vi "Grid_num_der.vi"(8 "error in (no error)":errorcluster, 9 "Settings":T1={"Cutoff frq I/V"=0.125, "Cutoff frq dI/dV"=0.125, "Filter order dI/DV"=2, "Filter type  dI/dV"=enum."Gaussian", "Filter order I/V"=2, "Filter type I/V"=enum."Gaussian"} {"Filter order I/V" min=1 max=1000 step=1; "Filter order dI/DV" min=1 max=1000 step=1}, 11 "Binary Spectroscopy File":path) -> (0 "error out":errorcluster)   [LabVIEW 2021]
uses:
  <userlib>/Nanonis Prog Interface V5/Nanonis Prog Interface.lvlib
panel:
  out "error out Write file":errorcluster
  out "error out Read file":errorcluster
  out "Progress":u8(slide) scale=0.0..100.0
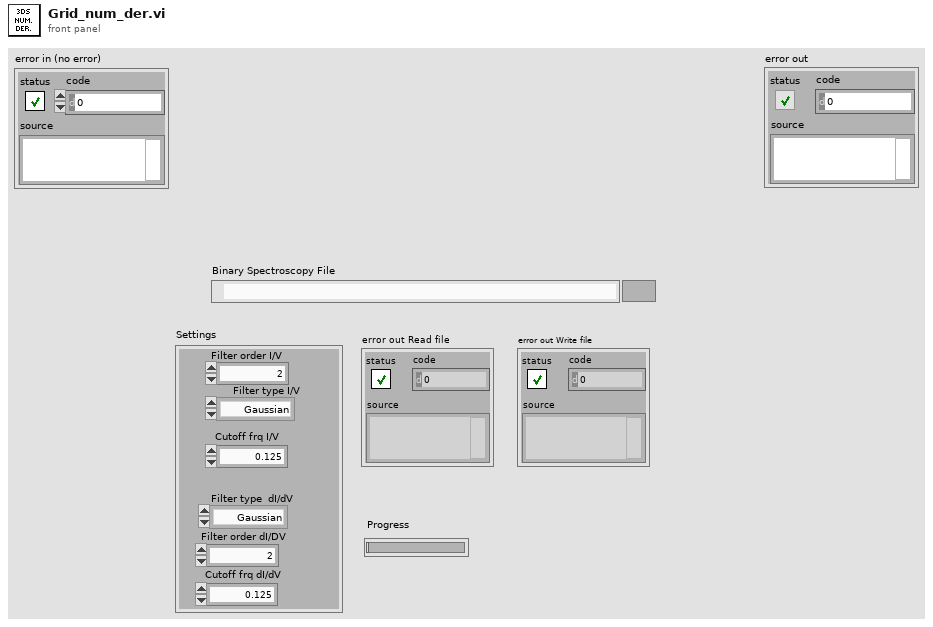
[diagram p1: front panel]
types:
  T1 = cluster{"Cutoff frq I/V":dbl, "Cutoff frq dI/dV":dbl, "Filter order dI/DV":i32, "Filter type  dI/dV":enum16{"none", "Gaussian", "Butterworth", "5th order FIR"}, "Filter order I/V":i32, "Filter type I/V":enum16{"none", "Gaussian", "Butterworth", "5th order FIR"}}
  T2 = typedef "Nanonis Prog Interface.lvlib/Binary_SpectroscopyFile-Config.ctl" = cluster{"Num Par":i32, "Exp size":i32, "Points":i32, "Grid Dim X":i32, "Grid Dim Y":i32, "Header size":i32, "Channels":string[], "Parameters":string[], "Sweep Signal":string, "Grid":cluster{"center X (m)":sgl, "center Y (m)":sgl, "width (m)":sgl, "height (m)":sgl, "angle (deg)":sgl}}
  T3 = cluster{"center X (m)":sgl, "center Y (m)":sgl, "width (m)":sgl, "height (m)":sgl, "angle (deg)":sgl}
  T4 = enum16{"none", "Gaussian", "Butterworth", "5th order FIR"}
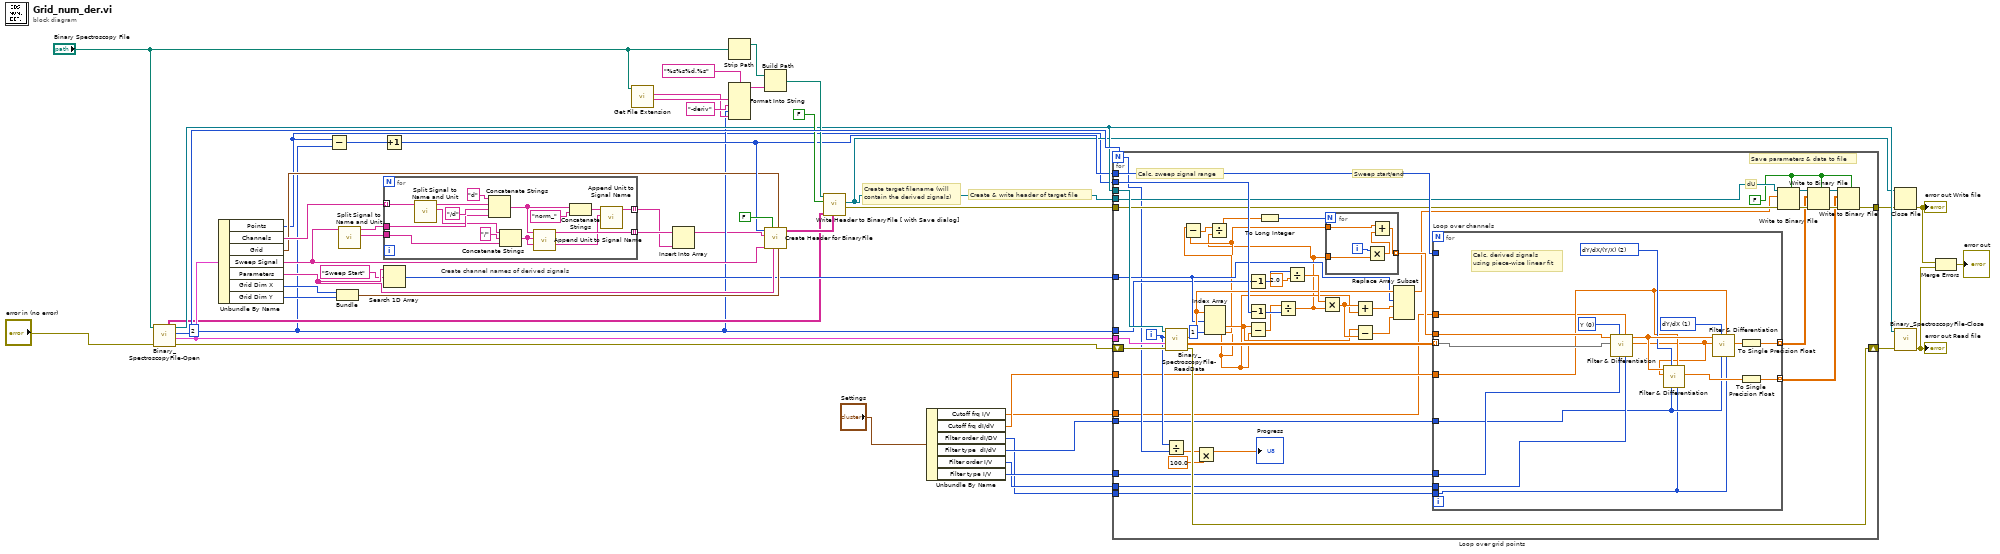
[diagram p0: block diagram]
diagram:
  w16 = u16 2 ("Fit length for derivative")
  # "Create & write header of target file"
  # "Create target filename (will contain the derived signals)"
  n1 = call <userlib>:"Binary_SpectroscopyFile-Open.vi"("error in (no error)"="error in (no error)", "Binary Spectroscopy File"="Binary Spectroscopy File") -> ("error out"=w48:errorcluster, "Config"=w36:T2, "Number of Experiments"=w49:i32, "File ref"=w37:refnum<file>, "Global Attributes"=w22:string[][])  [unwired: 5 in]
  n2 = Unbundle By Name(w36) -> ("Points"=w12:i32, "Channels"=w35:string[], "Grid"=w26:T3, "Sweep Signal"=w34:string, "Parameters"=w30:string[], "Grid Dim X"=w46:i32, "Grid Dim Y"=w45:i32)
  n3 = Subtract(x=w12, y=w16) -> (x-y=w31:i32)
  n4 = Bundle("Grid Dim X"=w46, "Grid Dim Y"=w45) -> (w44:cluster{"Grid Dim X":i32, "Grid Dim Y":i32})  [unwired: 1 in]
  n5 = call <userlib>:"Split Signal to Name and Unit.vi"("Name with unit"=w34) -> ("Unit"=w32:string, "Name"=w33:string)  [unwired: 5 in]
  n6 = Increment(x=w31) -> (x+1=w27:i32)
  n7 = for "Create channel names of derived signals" {
    tunnel: w35 -> [w63] mode=indexing
    tunnel: w33 -> [w59]
    tunnel: w32 -> [w56]
    tunnel: [w55] -> w14 mode=indexing
    tunnel: [w50] -> w13 mode=indexing
    n8 = call <userlib>:"Split Signal to Name and Unit.vi"("Name with unit"=w63) -> ("Unit"=w58:string, "Name"=w62:string)  [unwired: 5 in]
    n9 = Concatenate Strings("d" ("string"), w62, "/d" ("string"), w59) -> (w53:string)
    n10 = Concatenate Strings(w58, "/" ("string"), w56) -> (w54:string)
    n11 = call <userlib>:"Append Unit to Signal Name.vi"("Unit"=w54, "Name"=w53) -> ("Name with unit"=w55:string)  [unwired: 5 in]
    n12 = Concatenate Strings(w53, "norm_" ("string")) -> (w52:string)
    n13 = call <userlib>:"Append Unit to Signal Name.vi"("Unit"=w54, "Name"=w52) -> ("Name with unit"=w50:string)  [unwired: 5 in]
  }
  n14 = Search 1D Array(1D array=w30, element="Sweep Start") -> (index of element=w28:i32)  [unwired: 1 in]
  n15 = call <vilib>:"Get File Extension.vi"("file"="Binary Spectroscopy File") -> ("filename without extension"=w19:string, "lowercase file extension"=w18:string)  [unwired: 6 in, 3 out]
  n16 = Insert Into Array(array=w14, new element=w13) -> (w15:string[])  [unwired: 1 in]
  n17 = Strip Path(path="Binary Spectroscopy File") -> (stripped path=w42:path)  [unwired: 1 out]
  n18 = Format Into String(format string="%s%s%d.%s", w19, "-deriv" ("string"), w16, w18) -> (resulting string=w17:string)  [unwired: 2 in, 1 out]
  n19 = Build Path(base path=w42, name or relative path=w17) -> (appended path=w41:path)
  n20 = call <userlib>:"Create Header for BinaryFile.vi"("Grid points"=w44, "Grid param"=w26, "Fixed parameters"=w30, "Backward sweep"=FALSE, "Sweep signal"=w34, "Channels"=w15, "Points per sweep"=w27) -> ("Header (fixed attributes)"=w39:string[][])  [unwired: 4 in]
  n21 = call <userlib>:"Write Header to BinaryFile [ with Save dialog].vi"("Fixed Attributes"=w39, "Attributes in"=w22, "Show Dialog? (T)"=FALSE, "Filename"=w41) -> ("Error out"=w25:errorcluster, "File ref"=w23:refnum<file>)  [unwired: 4 in, 2 out]
  n22 = Unbundle By Name("Settings") -> ("Cutoff frq I/V"=w9:dbl, "Cutoff frq dI/dV"=w10:dbl, "Filter order dI/DV"=w5:i32, "Filter type  dI/dV"=w6:T4, "Filter order I/V"=w7:i32, "Filter type I/V"=w8:T4)
  n23 = for "Loop over grid points" {
    N: w49 -> [w72]
    tunnel: w37 -> [w112]
    tunnel: w36 -> [w111]
    shift-right: [w109] -> w38
    shift-left: w48 -> [w110]
    tunnel: w23 -> [w95]
    tunnel: w16 -> [w84]
    tunnel: w28 -> [w100]
    tunnel: w12 -> [w108]
    tunnel: w27 -> [w97]
    tunnel: w25 -> [w94]
    tunnel: [w91] -> w24
    tunnel: w10 -> [w69]
    tunnel: w9 -> [w68]
    tunnel: w8 -> [w67]
    tunnel: w7 -> [w66]
    tunnel: w6 -> [w65]
    tunnel: w5 -> [w64]
    i -> [w73]
    w88 = FALSE ("prepend array or string size? (T)")
    # "dU"
    # "Sweep start/end"
    # "Save parameters & data to file"
    # "Calc. sweep signal range"
    n24 = call <userlib>:"Binary_SpectroscopyFile-ReadData.vi"("error in"=w110, "Config"=w111, "Experiment to read (Index)"=w73, "File ref In"=w112) -> ("error out"=w109:errorcluster, "data"=w86:sgl[][], "Parameter values"=w101:sgl[])  [unwired: 4 in, 1 out]
    n25 = Divide(x=w73, y=w72) -> (x/y=w74:dbl)
    n26 = Multiply(x=w74, y=100.0) -> (x*y=→"Progress":dbl)
    n27 = Index Array(array=w101, index #1=w100, index #3=1 ("index")) -> (element #1=w79:sgl, element #2=w82:sgl, element #3=w80:sgl)  [unwired: 1 in]
    n28 = Subtract(x=w80, y=w79) -> (x-y=w78:sgl)
    n29 = Decrement(x=w84) -> (x-1=w105:u16)
    n30 = Decrement(x=w108) -> (x-1=w107:i32)
    n31 = Subtract(x=w82, y=w79) -> (x-y=w106:sgl)
    n32 = Divide(x=w106, y=w107) -> (x/y=w77:sgl)
    n33 = Divide(x=w78, y=w77) -> (x/y=w76:sgl)
    n34 = To Long Integer(number=w76) -> (32bit integer=w75:i32)
    n35 = Divide(x=w105, y=sgl 2.0) -> (x/y=w103:sgl)
    n36 = Multiply(x=w103, y=w77) -> (x*y=w102:sgl)
    n37 = for {
      N: w75 -> [_]
      tunnel: w77 -> [w116]
      tunnel: [w114] -> w96 mode=indexing
      tunnel: w79 -> [w113]
      i -> [w117]
      n38 = Multiply(x=w117, y=w116) -> (x*y=w115:sgl)
      n39 = Add(x=w113, y=w115) -> (x+y=w114:sgl)
    }
    n40 = Add(x=w102, y=w79) -> (x+y=w99:sgl)
    n41 = Subtract(x=w82, y=w102) -> (x-y=w98:sgl)
    n42 = Replace Array Subset(array=w101, new element #1=w99, index #1=w100, new element #2=w98) -> (w83:sgl[])  [unwired: 1 in]
    n43 = for "Loop over channels" {
      tunnel: w86 -> [w126] mode=indexing
      tunnel: w97 -> [_]
      tunnel: w96 -> [w134]
      tunnel: [w133] -> w89 mode=indexing
      tunnel: [w132] -> w85 mode=indexing
      tunnel: w69 -> [w125]
      tunnel: w68 -> [w124]
      tunnel: w67 -> [w123]
      tunnel: w66 -> [w122]
      tunnel: w65 -> [w121]
      tunnel: w64 -> [w120]
      w127 = u16 2 items=["Y", "dY/dX", "dY/dX/(Y/X)"] ("Display (Y)")
      w130 = u16 1 items=["Y", "dY/dX", "dY/dX/(Y/X)"] ("Display (Y)")
      w131 = u16 0 items=["Y", "dY/dX", "dY/dX/(Y/X)"] ("Display (Y)")
      # "Calc. derived signals using piece-wise linear fit"
      n44 = call <userlib>:"Filter & Differentiation.vi"("Filter order (2)"=w122, "Cutoff frq (0.125)"=w124, "Filter type (none)"=w123, "Display (Y)"=w131, "Y in"=w126, "X in"=w134) -> ("Y out"=w118:dbl[], "X out"=w129:dbl[])  [unwired: 3 in, 1 out]
      n45 = call <userlib>:"Filter & Differentiation.vi"("Filter order (2)"=w120, "Cutoff frq (0.125)"=w125, "Filter type (none)"=w121, "Display (Y)"=w127, "Y in"=w118, "X in"=w129) -> ("Y out"=w128:dbl[])  [unwired: 3 in, 2 out]
      n46 = call <userlib>:"Filter & Differentiation.vi"("Filter order (2)"=w120, "Cutoff frq (0.125)"=w125, "Filter type (none)"=w121, "Display (Y)"=w130, "Y in"=w118, "X in"=w129) -> ("Y out"=w119:dbl[])  [unwired: 3 in, 2 out]
      n47 = To Single Precision Float(number=w119) -> (single precision float=w133:sgl[])
      n48 = To Single Precision Float(number=w128) -> (single precision float=w132:sgl[])
    }
    n49 = Write to Binary File(file (use dialog)=w95, data=w83, error in=w94, 5:w88) -> (refnum out=w93:refnum<file>, error out=w92:errorcluster)  [unwired: 2 in, 1 out]
    n50 = Write to Binary File(file (use dialog)=w93, data=w89, error in=w92, 5:w88) -> (refnum out=w87:refnum<file>, error out=w90:errorcluster)  [unwired: 2 in, 1 out]
    n51 = Write to Binary File(file (use dialog)=w87, data=w85, error in=w90, 5:w88) -> (error out=w91:errorcluster)  [unwired: 2 in, 2 out]
  }
  n52 = Close File(refnum=w23, error in=w24) -> (error out=w4:errorcluster)  [unwired: 1 out]
  "error out Write file" <- w4
  n53 = call <userlib>:"Binary_SpectroscopyFile-Close.vi"("error in"=w38, "File ref"=w37) -> ("error out"=w3:errorcluster)  [unwired: 9 in]
  "error out Read file" <- w3
  n54 = Merge Errors(w4, w3) -> (→"error out":errorcluster)
